vi "ASK.vi"() -> ()   [LabVIEW 2015]
panel:
  out "Waveform Graph":dbl[](graph)=[0.0, 0.9510565162951535, 0.5877852522924732, -0.5877852522924734, -0.9510565162951536, -2.4492935982947064e-16, 0.9510565162951538, 0.5877852522924734, -0.5877852522924728, -0.9510565162951538, -4.898587196589413e-16, 0.951056516295154, 0.5877852522924721, 0.0, 0.0, 0.0, -0.0, -0.0, 0.0, 0.0, 0.0, -0.0, -0.0, 0.0, 0.0, 0.0, 0.9510565162951532, 0.5877852522924742, -0.587785252292472, -0.9510565162951519, -1.4695761589768238e-15, 0.9510565162951531, 0.5877852522924744, -0.5877852522924718, -0.9510565162951519, -1.7145055188062944e-15, 0.951056516295153, 0.5877852522924746, 0.0, 0.0, 0.0, -0.0, -0.0, 0.0, 0.0, 0.0, -0.0, -0.0, 0.0, 0.0, 0.0, 0.951056516295155, 0.5877852522924751, -0.5877852522924768, -0.9510565162951544, -9.799650315725178e-15, 0.9510565162951528, 0.5877852522924696, -0.5877852522924824, -0.9510565162951523, -2.9391523179536475e-15, 0.9510565162951549, 0.5877852522924756, 0.0, 0.0, -0.0, -0.0, -0.0, 0.0, 0.0, 0.0, -0.0, -0.0, 0.0, 0.0, 0.0, 0.9510565162951524, 0.5877852522924705, -0.5877852522924816, -0.9510565162951525]
  out "Modulating wave 2":dbl[](graph)=[0.0, 0.9510565162951535, 0.5877852522924732, -0.5877852522924734, -0.9510565162951536, -2.4492935982947064e-16, 0.9510565162951538, 0.5877852522924734, -0.5877852522924728, -0.9510565162951538, -4.898587196589413e-16, 0.951056516295154, 0.5877852522924721, -0.5877852522924726, -0.9510565162951538, -7.347880794884119e-16, 0.9510565162951533, 0.5877852522924709, -0.5877852522924724, -0.9510565162951539, -9.797174393178826e-16, 0.9510565162951533, 0.5877852522924711, -0.5877852522924751, -0.9510565162951529, -1.2246467991473533e-15, 0.9510565162951532, 0.5877852522924742, -0.587785252292472, -0.9510565162951519, -1.4695761589768238e-15, 0.9510565162951531, 0.5877852522924744, -0.5877852522924718, -0.9510565162951519, -1.7145055188062944e-15, 0.951056516295153, 0.5877852522924746, -0.5877852522924716, -0.951056516295152, -1.959434878635765e-15, 0.9510565162951552, 0.5877852522924748, -0.5877852522924714, -0.9510565162951521, -2.204364238465236e-15, 0.9510565162951551, 0.587785252292475, -0.587785252292477, -0.9510565162951521, -2.4492935982947065e-15, 0.951056516295155, 0.5877852522924751, -0.5877852522924768, -0.9510565162951544, -9.799650315725178e-15, 0.9510565162951528, 0.5877852522924696, -0.5877852522924824, -0.9510565162951523, -2.9391523179536475e-15, 0.9510565162951549, 0.5877852522924756, -0.5877852522924764, -0.9510565162951545, 3.921345679817883e-15, 0.9510565162951525, 0.58778525229247, -0.5877852522924819, -0.9510565162951524, -3.429011037612589e-15, 0.9510565162951546, 0.587785252292476, -0.587785252292476, -0.9510565162951546, -1.0779367755043061e-14, 0.9510565162951524, 0.5877852522924705, -0.5877852522924816, -0.9510565162951525]
  out "Numeric 2":dbl=-1.1882855810441129e-16
  in  "phase 2":dbl
  in  "Amplitude 2":dbl=1.0
  in  "Fs 2":dbl=500.0
  in  "Frequency 2":dbl=100.0
  in  "No of Iteration 2":i32=80
  out "Modulating wave":dbl[](graph)=[0.0, 1.0, 1.0, 1.0, 1.0, 1.0, 1.0, 1.0, 1.0, 1.0, 1.0, 1.0, 1.0, -0.0, -0.0, -0.0, -0.0, -0.0, -0.0, -0.0, -0.0, -0.0, -0.0, -0.0, -0.0, -0.0, 1.0, 1.0, 1.0, 1.0, 1.0, 1.0, 1.0, 1.0, 1.0, 1.0, 1.0, 1.0, -0.0, -0.0, -0.0, -0.0, -0.0, -0.0, -0.0, -0.0, -0.0, -0.0, -0.0, -0.0, -0.0, 1.0, 1.0, 1.0, 1.0, 1.0, 1.0, 1.0, 1.0, 1.0, 1.0, 1.0, 1.0, -0.0, -0.0, -0.0, -0.0, -0.0, -0.0, -0.0, -0.0, -0.0, -0.0, -0.0, -0.0, -0.0, 1.0, 1.0, 1.0, 1.0]
  out "Numeric":dbl=0.0045186371853945355
  in  "phase":dbl
  in  "Amplitude":dbl=1.0
  in  "Fs":dbl=500.0
  in  "Frequency":dbl=20.0
  in  "No of Iteration":i32=80
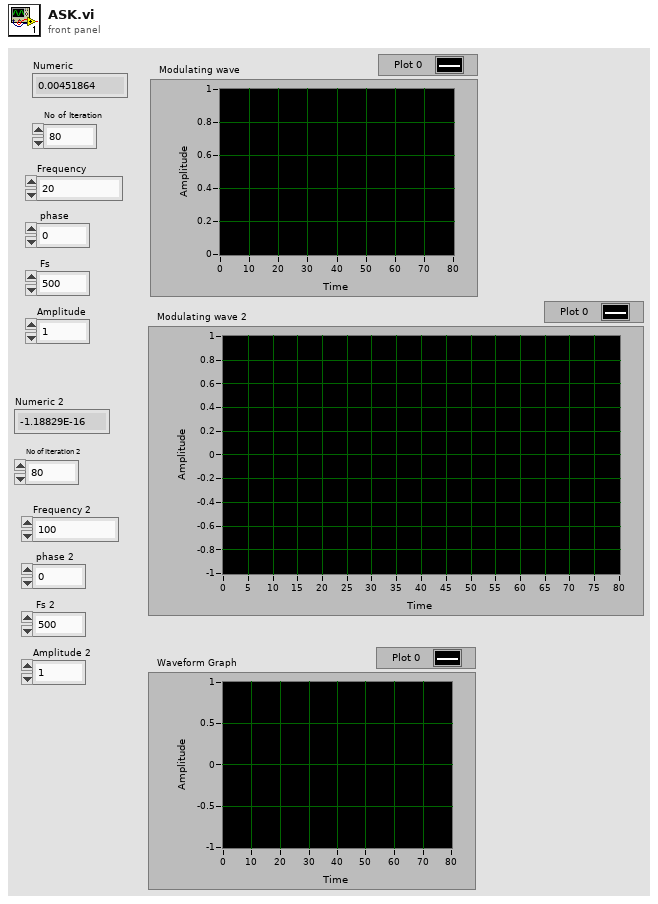
[diagram p1: front panel]
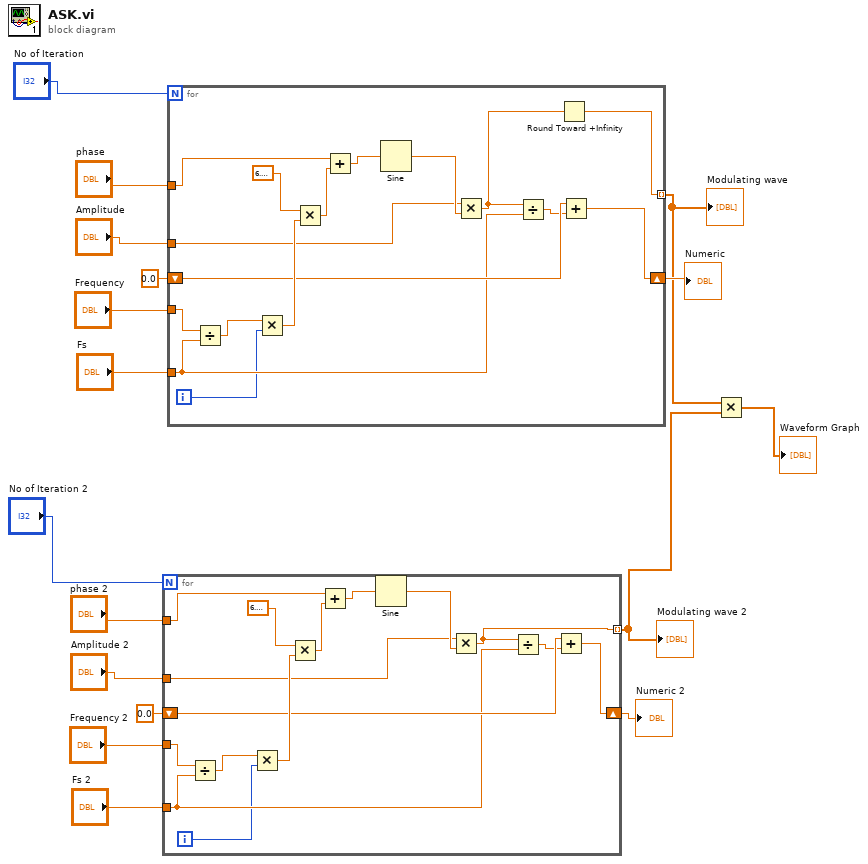
[diagram p0: block diagram]
diagram:
  n1 = for {
    N: "No of Iteration 2" -> [_]
    tunnel: "Frequency 2" -> [w31]
    tunnel: "Fs 2" -> [w21]
    tunnel: "Amplitude 2" -> [w27]
    tunnel: "phase 2" -> [w26]
    shift-right: [w20] -> w5
    shift-left: 0.0 -> [w24]
    tunnel: [w19] -> w3 mode=indexing
    i -> [w18]
    n2 = Divide(x=w31, y=w21) -> (x/y=w25:dbl)
    n3 = Multiply(x=w25, y=w18) -> (x*y=w29:dbl)
    n4 = Multiply(x=6.283185307179586, y=w29) -> (x*y=w30:dbl)
    n5 = Add(x=w26, y=w30) -> (x+y=w32:dbl)
    n6 = Sine(x=w32) -> (sin(x)=w28:dbl)
    n7 = Multiply(x=w27, y=w28) -> (x*y=w19:dbl)
    n8 = Divide(x=w19, y=w21) -> (x/y=w22:dbl)
    n9 = Add(x=w24, y=w22) -> (x+y=w20:dbl)
  }
  "Numeric 2" <- w5
  "Modulating wave 2" <- w3
  n10 = for {
    N: "No of Iteration" -> [_]
    tunnel: "Frequency" -> [w47]
    tunnel: "Fs" -> [w37]
    tunnel: "Amplitude" -> [w43]
    tunnel: "phase" -> [w42]
    shift-right: [w33] -> w12
    shift-left: 0.0 -> [w40]
    tunnel: [w35] -> w2 mode=indexing
    i -> [w36]
    n11 = Divide(x=w47, y=w37) -> (x/y=w41:dbl)
    n12 = Multiply(x=w41, y=w36) -> (x*y=w45:dbl)
    n13 = Multiply(x=6.283185307179586, y=w45) -> (x*y=w46:dbl)
    n14 = Add(x=w42, y=w46) -> (x+y=w48:dbl)
    n15 = Sine(x=w48) -> (sin(x)=w44:dbl)
    n16 = Multiply(x=w43, y=w44) -> (x*y=w34:dbl)
    n17 = Divide(x=w34, y=w37) -> (x/y=w38:dbl)
    n18 = Round Toward +Infinity(x=w34) -> (ceil(x): smallest int >= x=w35:dbl)
    n19 = Add(x=w40, y=w38) -> (x+y=w33:dbl)
  }
  "Numeric" <- w12
  "Modulating wave" <- w2
  n20 = Multiply(x=w2, y=w3) -> (x*y=→"Waveform Graph":dbl[])
